vi "Write No Error.vi"(7 "Ignore Network Down":bool, 8 "error in (no error)":errorcluster) -> (0 "error out":errorcluster, 6 "Comm Error":bool)   [LabVIEW 2011]
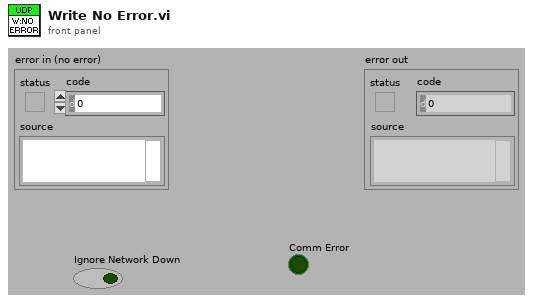
[diagram p1: front panel]
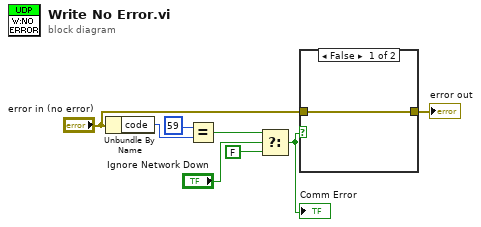
[diagram p0: block diagram]
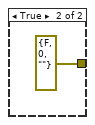
[diagram p2: hidden frame]
diagram:
  n1 = Unbundle By Name("error in (no error)") -> ("code"=w8:i32)
  n2 = Equal?(x=59, y=w8) -> (x = y?=w6:bool)
  n3 = Select(t=w6, s="Ignore Network Down", f=FALSE) -> (s? t:f=w1:bool)
  "Comm Error" <- w1
  n4 = case shown="False" w1 {
    tunnel: "error in (no error)" -> [w9 _]
    tunnel: [w9 errorcluster {"status"=FALSE, "code"=0, "source"=""} ("error out")] -> w3
    frame False {
    }
    frame True {
    }
  }
  "error out" <- w3
